vi "users delete user.vi"(6 "Current User (none)":T1, 8 "error in (no error)":errorcluster, 10 "Username (\"\")":string, 11 "Connection Refnum":T2) -> (0 "error out":errorcluster, 3 "Connection Refnum":T2)   [LabVIEW 2011]
uses:
  Summitek EXT/ODBC/SQL Controls/Connection Refnum.ctl
  server/database/Users/User Record.ctl
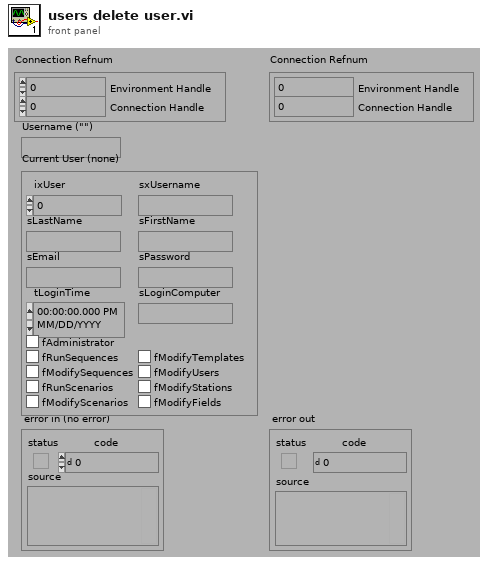
[diagram p1: front panel]
types:
  T1 = typedef "User Record.ctl" = cluster{"ixUser":i32, "sxUsername":string, "sLastName":string, "sFirstName":string, "sEmail":string, "sPassword":string, "tLoginTime":timestamp, "sLoginComputer":string, "fAdministrator":bool, "fRunSequences":bool, "fModifySequences":bool, "fRunScenarios":bool, "fModifyScenarios":bool, "fModifyTemplates":bool, "fModifyUsers":bool, "fModifyStations":bool, "fModifyFields":bool}
  T2 = typedef "Connection Refnum.ctl" = cluster{"Environment Handle":i32, "Connection Handle":i32}
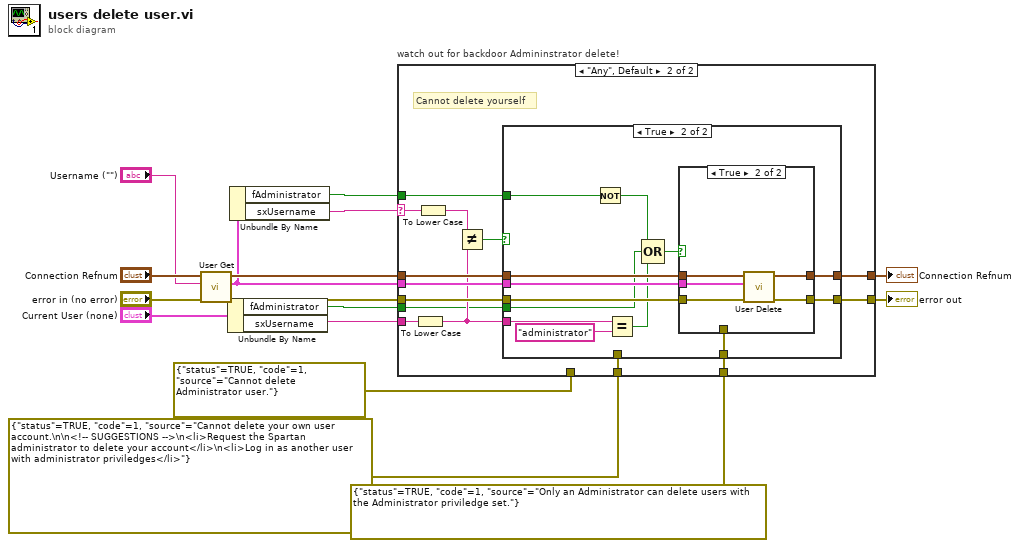
[diagram p0: block diagram]
diagram:
  n1 = call "User Get.vi"("error in (no error)"="error in (no error)", "sxUsername (\"\")"="Username (\"\")", "Connection Refnum"="Connection Refnum") -> ("error out"=w16:errorcluster, "User"=w13:T1, "Connection Refnum"=w15:T2)  [unwired: 6 out]
  n2 = Unbundle By Name("Current User (none)") -> ("fAdministrator"=w1:bool, "sxUsername"=w4:string)
  n3 = Unbundle By Name(w13) -> ("fAdministrator"=w2:bool, "sxUsername"=w12:string)
  n4 = case "watch out for backdoor Admininstrator delete!" shown="\"Any\", Default" w12 {
    selector: w12 -> [_ w27]
    tunnel: [w17 w32] -> w10
    tunnel: w16 -> [_ w31]
    tunnel: w15 -> [w18 w30]
    tunnel: [w18 w29] -> w9
    tunnel: w13 -> [_ w28]
    tunnel: errorcluster {"status"=TRUE, "code"=1, "source"="Cannot delete your own user account.\n\n<!-- SUGGESTIONS -->\n<li>Request the Spartan administrator to delete your account</li>\n<li>Log in as another user with administrator priviledges</li>"} ("error out") -> [_ w24]
    tunnel: errorcluster {"status"=TRUE, "code"=1, "source"="Cannot delete Administrator user."} ("error out") -> [w17 _]
    tunnel: w4 -> [_ w23]
    tunnel: errorcluster {"status"=TRUE, "code"=1, "source"="Only an Administrator can delete users with the Administrator priviledge set."} ("error out") -> [_ w22]
    tunnel: w2 -> [_ w20]
    tunnel: w1 -> [_ w19]
    frame "administrator" {
    }
    frame "Any", Default {
      # "Cannot delete yourself"
      n5 = To Lower Case(string=w23) -> (all lower case string=w21:string)
      n6 = To Lower Case(string=w27) -> (all lower case string=w26:string)
      n7 = Not Equal?(x=w26, y=w21) -> (x != y?=w25:bool)
      n8 = case shown="True" w25 {
        tunnel: [w33 w47] -> w32
        tunnel: w31 -> [_ w46]
        tunnel: w30 -> [w34 w45]
        tunnel: [w34 w44] -> w29
        tunnel: w28 -> [_ w43]
        tunnel: w24 -> [w33 _]
        tunnel: w22 -> [_ w36]
        tunnel: w21 -> [_ w41]
        tunnel: w20 -> [_ w39]
        tunnel: w19 -> [_ w35]
        frame False {
        }
        frame True {
          n9 = Not(x=w39) -> (.not. x?=w38:bool)
          n10 = Equal?(x=w41, y="administrator") -> (x = y?=w40:bool)
          n11 = Compound Arithmetic op=OR(w38, w35, w40) -> (w37:bool)
          n12 = case shown="True" w37 {
            tunnel: [w49 w54] -> w47
            tunnel: w46 -> [_ w53]
            tunnel: w45 -> [w48 w52]
            tunnel: [w48 w51] -> w44
            tunnel: w43 -> [_ w50]
            tunnel: w36 -> [w49 _]
            frame False {
            }
            frame True {
              n13 = call "User Delete.vi"("error in (no error)"=w53, "User Record"=w50, "Connection Refnum"=w52) -> ("error out"=w54:errorcluster, "Connection Refnum"=w51:T2)  [unwired: 7 out]
            }
          }
        }
      }
    }
  }
  "error out" <- w10
  "Connection Refnum" <- w9
